vi "Chart Display Size.vi"() -> ()   [LabVIEW 2011]
panel:
  in  "Values to Display":dbl=100.0
  in  "Stop Button":bool
  out "Waveform Chart":cluster{dbl, dbl}(graph)={7.956691168296501, 6.365352934637201}
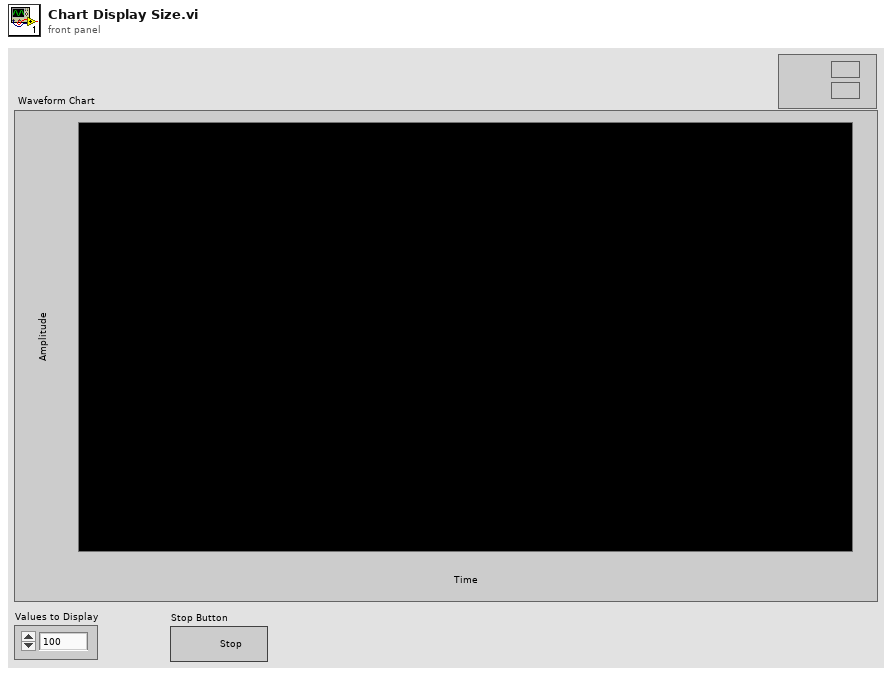
[diagram p1: front panel]
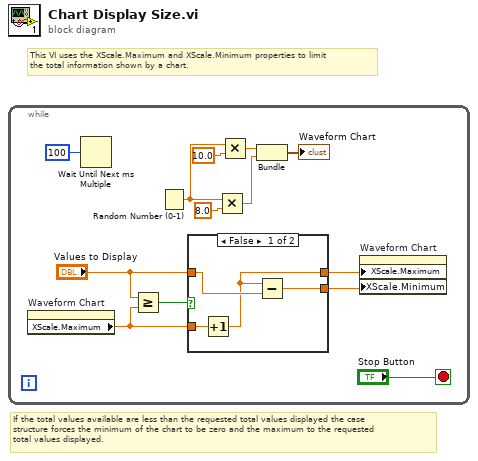
[diagram p0: block diagram]
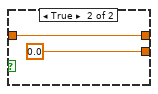
[diagram p2: hidden frame]
diagram:
  # "If the total values available are less than the requested total values displayed the case\nstructure forces the minimum of the chart to be zero and the maximum to the requested\ntotal values displayed."
  # "This VI uses the XScale.Maximum and XScale.Minimum properties to limit \nthe total information shown by a chart."
  n1 = while {
    stop <- "Stop Button" stop-if-true
    n2 = property on="Waveform Chart" class="WFChart (strict)"() -> ("XScale.Maximum"=w1:dbl)  [unwired: 2 in, 2 out]
    n3 = Wait Until Next ms Multiple(millisecond multiple=u32 100) -> ()  [unwired: 1 out]
    n4 = Greater Or Equal?(x="Values to Display", y=w1) -> (x >= y?=w2:bool)
    n5 = Random Number (0-1)() -> (number: 0 to 1=w10:dbl)
    n6 = case shown="False" w2 {
      tunnel: "Values to Display" -> [w15 w19]
      tunnel: w1 -> [w17 _]
      tunnel: [w14 w19] -> w4
      tunnel: [w16 0.0] -> w5
      frame False {
        n7 = Increment(x=w17) -> (x+1=w14:dbl)
        n8 = Subtract(x=w14, y=w15) -> (x-y=w16:dbl)
      }
      frame True {
      }
    }
    n9 = Multiply(x=w10, y=8.0) -> (x*y=w7:dbl)
    n10 = Multiply(x=w10, y=10.0) -> (x*y=w6:dbl)
    n11 = Bundle(w6, w7) -> (→"Waveform Chart":cluster{dbl, dbl})  [unwired: 1 in]
    n12 = property on="Waveform Chart" class="WFChart (strict)"("XScale.Maximum"=w4, "XScale.Minimum"=w5) -> ()  [unwired: 2 in, 2 out]
  }
